vi "readMatFileToNx1Array.vi"(8 "error in (no error)":errorcluster, 9 "Index of Column":i32[](array[numeric]), 10 "Index of Row":i32[](array[numeric]), 11 "Path":path) -> (0 "error out":errorcluster, 2 "nx1 Array":dbl[][](array[numeric]))   [LabVIEW 2016]
doc: "Read the 2D matrix file and transform to nx1 array based on the index of row and column."
uses:
  getSubArray2D.vi
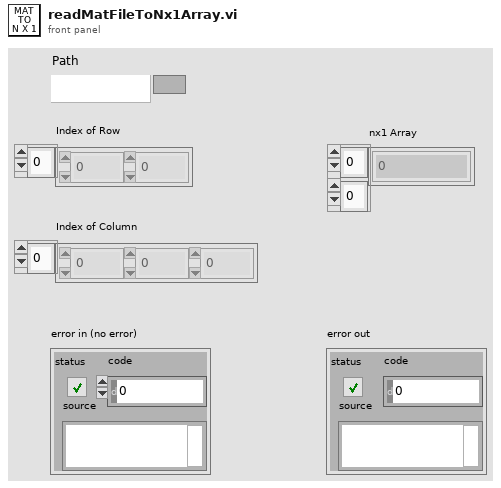
[diagram p1: front panel]
types:
  T1 = cluster{"Index of Row":i32[], "Index of Column":i32[]}
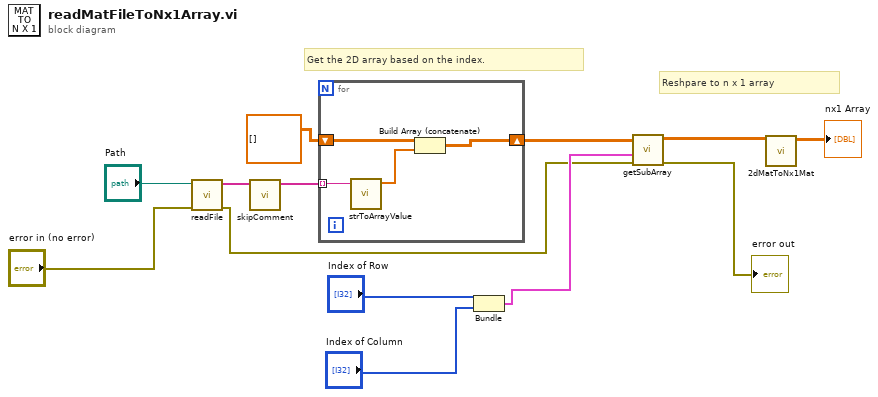
[diagram p0: block diagram]
diagram:
  # "Reshpare to n x 1 array"
  # "Get the 2D array based on the index."
  n1 = call "readFile.vi"("error in (no error)"="error in (no error)", "Path"="Path") -> ("error out"=w4:errorcluster, "Array"=w11:string[])  [unwired: 8 in]
  n2 = call "skipComment.vi"("Content"=w11) -> ("Content without Comment"=w9:string[])  [unwired: 10 in]
  n3 = for {
    tunnel: w9 -> [w17] mode=indexing
    shift-right: [w14] -> w1
    shift-left: dbl[][] [] -> [w15]
    n4 = call "strToArrayValue.vi"("String"=w17) -> ("Array"=w16:dbl[])  [unwired: 10 in]
    n5 = Build Array (concatenate)(w15, w16) -> (w14:dbl[][])
  }
  n6 = Bundle("Index of Row"="Index of Row", "Index of Column"="Index of Column") -> (w5:T1)  [unwired: 1 in]
  n7 = call-poly "getSubArray.vi"("error in (no error)"=w4, "Index Array Cluster"=w5, "2D Array"=w1) -> ("error out"=→"error out":errorcluster, "Sub-Array"=w2:dbl[][])  [unwired: 7 in]
  n8 = call "2dMatToNx1Mat.vi"("2D Array"=w2) -> ("nx1 Array"=→"nx1 Array":dbl[][])  [unwired: 10 in]
